vi "Check Close.vi"(11 "Sequence in":refnum<class "Sequence.lvclass">) -> (2 "Close":bool)   [LabVIEW 2020, in "VolatusSeq.lvlib" / "Sequence.lvclass"]
uses:
  Sequence.lvclass
  Sequence.lvclass/Sequence.ctl
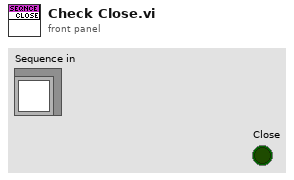
[diagram p1: front panel]
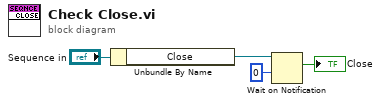
[diagram p0: block diagram]
diagram:
  n1 = Unbundle By Name("Sequence in") -> ("Close"=w3:refnum<notifier>)
  n2 = Wait on Notification(notifier=w3, timeout in ms (-1)=0) -> (notification=→"Close":bool)  [unwired: 2 in, 3 out]
